vi "Finalize.vi"(8 "Error in":errorcluster, 10 "Msg Output":refnum<class "Msg Output.lvclass">, 11 "TEMPLATE Actor in":refnum<class "TEMPLATE Actor.lvclass">) -> (0 "Error out":errorcluster, 3 "TEMPLATE Actor out":refnum<class "TEMPLATE Actor.lvclass">)   [LabVIEW 2020, in "_Template.lvlib" / "Templates.lvlib" / "TEMPLATE jettl Actor.lvlib" / "TEMPLATE Actor.lvlib" / "TEMPLATE Actor.lvclass"]
uses:
  TEMPLATE Actor.lvclass
  C:/git/jettl/src/jettl/jettl/Actor/Actor.lvclass
  jettl/jettl/Msg Output/Msg Output.lvclass
  jettl/jettl/Actor/Actor.lvclass
  TEMPLATE Actor.lvclass/TEMPLATE Actor.ctl
  jettl/jettl/jettl.lvlib
panel:
  # "This front panel should not be manipulated."
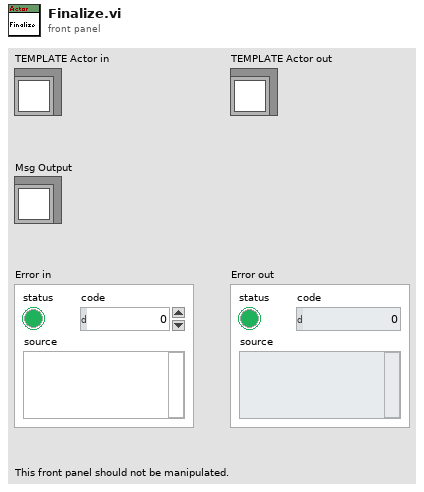
[diagram p1: front panel]
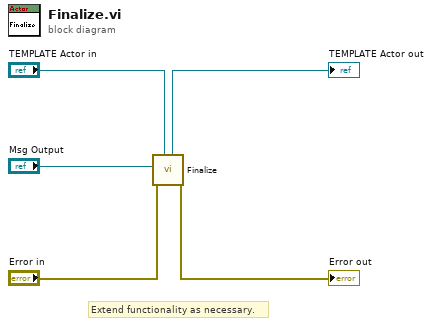
[diagram p0: block diagram]
diagram:
  # "Extend functionality as necessary."
  n1 = call "Finalize.vi"("Actor in"="TEMPLATE Actor in", "Error in"="Error in", "Msg Output"="Msg Output") -> ("Error out"=→"Error out":errorcluster, "Actor out"=→"TEMPLATE Actor out":refnum<class "TEMPLATE Actor.lvclass">)  [unwired: 7 in]
